vi "[Global] ItemNames.vi"() -> ()   [LabVIEW 2019]
panel:
  out "Item Names":string[][](array[string])
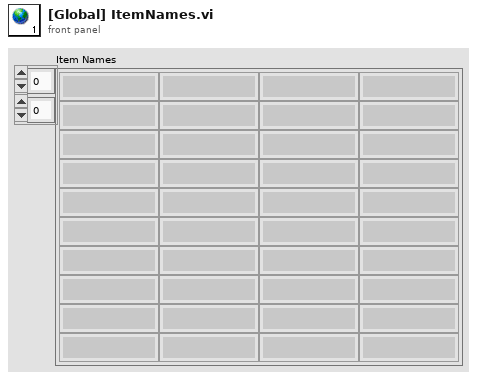
[diagram p1: front panel]
diagram:
